vi "state run pump.vi"(6 "pump command":T1, 7 "State":i16) -> (0 "rpm":dbl, 1 "registers":u16[](array[numeric]), 2 "run pump":bool, 3 "0, 1":i16)   [LabVIEW 2015]
uses:
  ProgramData/ProCoDA/Functions/Modbus devices/Pump.ctl
panel:
  out "array of states":u8[](array[numeric])
  out "data string":string
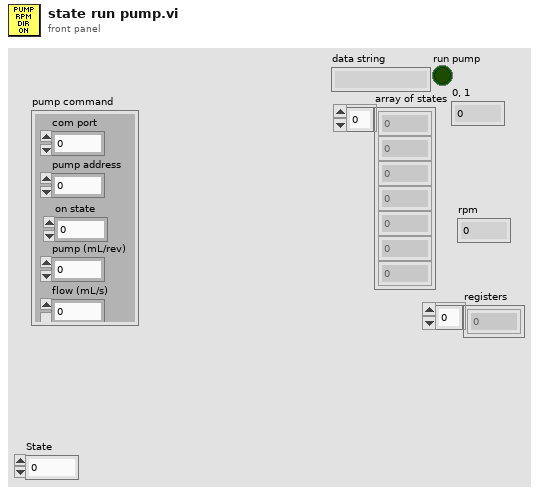
[diagram p1: front panel]
types:
  T1 = typedef "Pump.ctl" = cluster{"com port":u8, "pump address":u8, "on state":i32, "pump (mL/rev)":dbl, "flow (mL/s)":dbl}
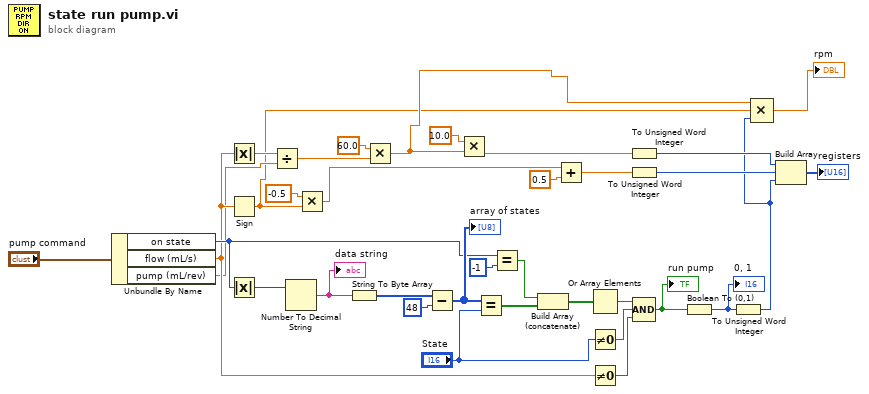
[diagram p0: block diagram]
diagram:
  n1 = Unbundle By Name("pump command") -> ("on state"=w30:i32, "flow (mL/s)"=w15:dbl, "pump (mL/rev)"=w14:dbl)
  n2 = Absolute Value(x=w15) -> (abs(x)=w18:dbl)
  n3 = Sign(1:w15) -> (0:w1:dbl)
  n4 = Absolute Value(x=w30) -> (abs(x)=w25:i32)
  n5 = Divide(x=w18, y=w14) -> (x/y=w20:dbl)
  n6 = Number To Decimal String(number=w25) -> (decimal integer string=w35:string)  [unwired: 1 in]
  "data string" <- w35
  n7 = Multiply(x=-0.5, y=w1) -> (x*y=w17:dbl)
  n8 = String To Byte Array(string=w35) -> (unsigned byte array=w34:u8[])
  n9 = Multiply(x=60.0, y=w20) -> (x*y=w5:dbl)
  n10 = Subtract(x=w34, y=48) -> (x-y=w32:i32[])
  "array of states" <- w32
  n11 = Multiply(x=10.0, y=w5) -> (x*y=w7:dbl)
  n12 = Equal?(x=w32, y="State") -> (x = y?=w28:bool[])
  n13 = Equal?(x=w30, y=-1) -> (x = y?=w27:bool)
  n14 = Build Array (concatenate)(w27, w28) -> (w26:bool[])
  n15 = Add(x=w17, y=0.5) -> (x+y=w4:dbl)
  n16 = Or Array Elements(Boolean array=w26) -> (logical OR=w24:bool)
  n17 = Not Equal To 0?(x="State") -> (x != 0?=w23:bool)
  n18 = Not Equal To 0?(x=w15) -> (x != 0?=w21:bool)
  n19 = To Unsigned Word Integer(number=w7) -> (unsigned 16bit integer=w12:u16)
  n20 = To Unsigned Word Integer(number=w4) -> (unsigned 16bit integer=w11:u16)
  n21 = Compound Arithmetic op=AND(w24, w23, w21) -> (w22:bool)
  "run pump" <- w22
  n22 = Boolean To (0,1)(Boolean=w22) -> (0, 1=w10:i16)
  "0, 1" <- w10
  n23 = To Unsigned Word Integer(number=w10) -> (unsigned 16bit integer=w3:u16)
  n24 = Compound Arithmetic op=MULTIPLY(w5, w1, w3) -> (→"rpm":dbl)
  n25 = Build Array(w12, w11, w3) -> (→"registers":u16[])
